vi "make_reg_config_ASIC.vi"(1 "Ib_ClipVb":u32, 2 "Clip_sel_b":u32, 3 "Att_en_b":bool, 4 "Clip_en_b":bool, 5 "CompBuf_en_b":bool, 6 "Att gain":u32) -> (0 "Out reg value":u32 format="%x")   [LabVIEW 2012]
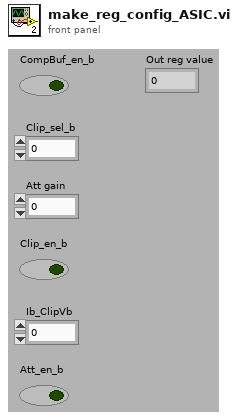
[diagram p1: front panel]
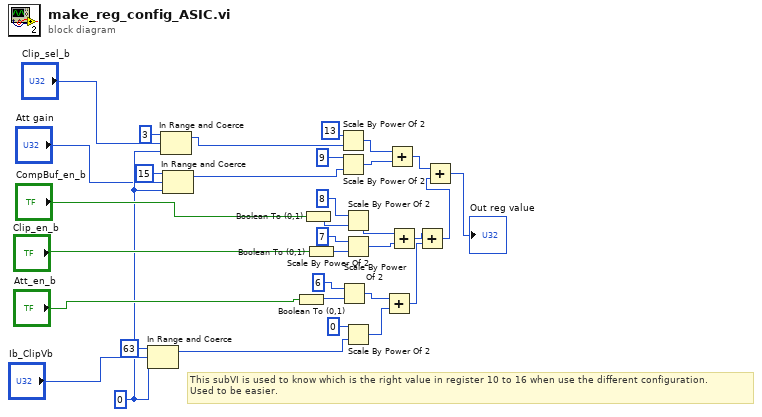
[diagram p0: block diagram]
diagram:
  w6 = u32 0 ("lower limit")
  # "This subVI is used to know which is the right value in register 10 to 16 when use the different configuration.\nUsed to be easier."
  n1 = In Range and Coerce(upper limit=u32 63, x="Ib_ClipVb", lower limit=w6) -> (coerced(x)=w7:u32)  [unwired: 1 out]
  n2 = In Range and Coerce(upper limit=u32 3, x="Clip_sel_b", lower limit=w6) -> (coerced(x)=w9:u32)  [unwired: 1 out]
  n3 = In Range and Coerce(upper limit=u32 15, x="Att gain", lower limit=w6) -> (coerced(x)=w4:u32)  [unwired: 1 out]
  n4 = Boolean To (0,1)(Boolean="Att_en_b") -> (0, 1=w26:i16)
  n5 = Boolean To (0,1)(Boolean="CompBuf_en_b") -> (0, 1=w28:i16)
  n6 = Boolean To (0,1)(Boolean="Clip_en_b") -> (0, 1=w27:i16)
  n7 = Scale By Power Of 2(n=13, x=w9) -> (x*2^n=w15:u32)
  n8 = Scale By Power Of 2(n=9, x=w4) -> (x*2^n=w16:u32)
  n9 = Scale By Power Of 2(n=6, x=w26) -> (x*2^n=w29:i16)
  n10 = Scale By Power Of 2(n=8, x=w28) -> (x*2^n=w20:i16)
  n11 = Scale By Power Of 2(n=7, x=w27) -> (x*2^n=w21:i16)
  n12 = Scale By Power Of 2(n=0, x=w7) -> (x*2^n=w13:u32)
  n13 = Add(x=w29, y=w13) -> (x+y=w23:u32)
  n14 = Add(x=w15, y=w16) -> (x+y=w25:u32)
  n15 = Add(x=w20, y=w21) -> (x+y=w22:i16)
  n16 = Add(x=w22, y=w23) -> (x+y=w24:u32)
  n17 = Add(x=w25, y=w24) -> (x+y=→"Out reg value":u32)
